vi "SquareFilter1.vi"(3 "error IN":errorcluster, 4 "Areas":dbl[][](array[numeric]), 5 "X,Y":dbl[][](array[numeric]), 6 "[IN] Chains (X,Y,dX,dY)":dbl[][](array[numeric])) -> (0 "error OUT":errorcluster, 2 "Filtered Chains (X,Y,dX,dY)":dbl[][](array[numeric]))   [LabVIEW 2013]
doc: "This simple filter cuts out displacement which connects particles with relative difference in areas more than 50%"
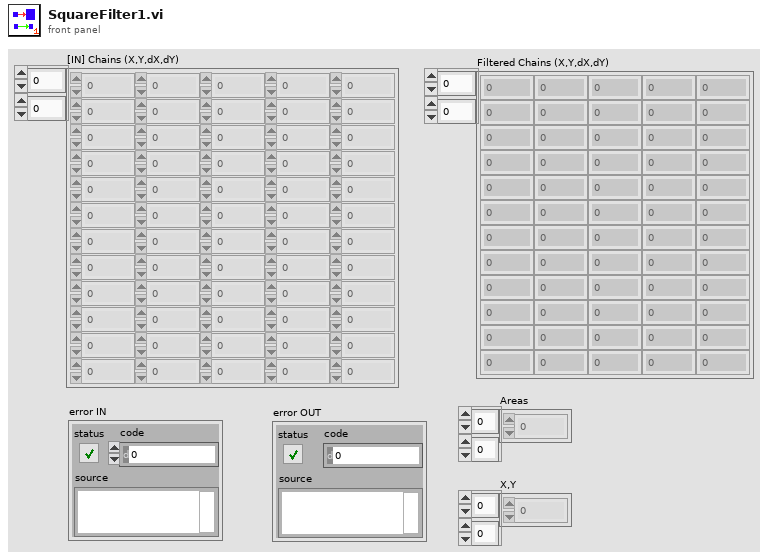
[diagram p1: front panel]
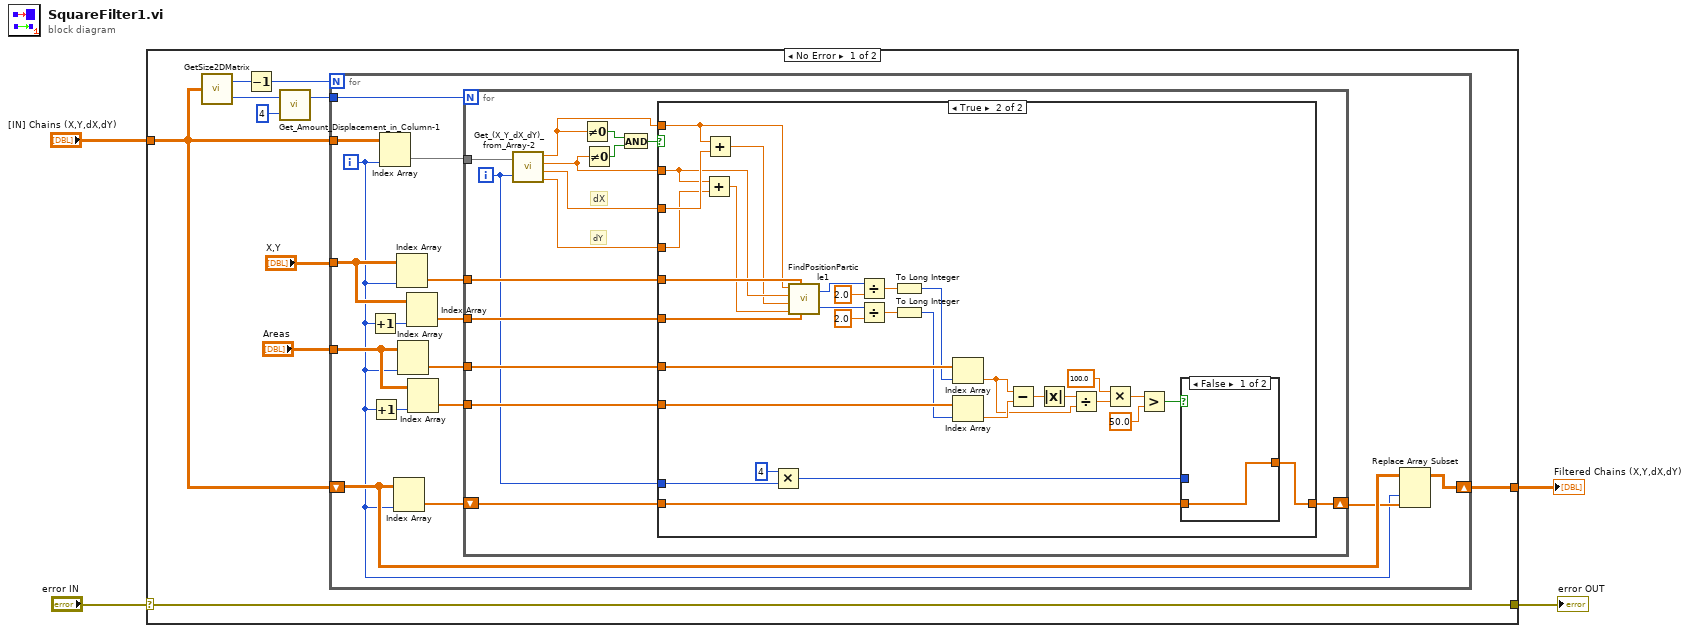
[diagram p0: block diagram]
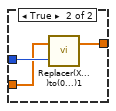
[diagram p3: hidden frame]
diagram:
  n1 = case shown="No Error" "error IN" {
    selector: "error IN" -> [w5 w83]
    tunnel: [w14 w84] -> w4
    tunnel: "[IN] Chains (X,Y,dX,dY)" -> [w10 w84]
    tunnel: [w5 w83] -> w1
    frame No Error {
      n2 = call "GetSize2DMatrix.vi"("Array IN (2D)"=w10) -> ("# Cols"=w9:i32, "# Rows"=w7:i32)
      n3 = Decrement(x=w9) -> (x-1=w13:i32)
      n4 = call "Get_Amount_Displacement_in_Column-1.vi"("multiplier"=4, "# Rows"=w7) -> ("Displ amount"=w6:i32)  [unwired: 1 out]
      n5 = for {
        N: w13 -> [_]
        tunnel: w10 -> [w29]
        shift-right: [w17] -> w14
        shift-left: w10 -> [w19]
        tunnel: "Areas" -> [w23]
        tunnel: "X,Y" -> [w28]
        tunnel: w6 -> [w15]
        i -> [w16]
        n6 = Increment(x=w16) -> (x+1=w27:i32)
        n7 = Increment(x=w16) -> (x+1=w24:i32)
        n8 = Index Array(array=w29, index (col)=w16) -> (element=w30:dbl[])  [unwired: 1 in]
        n9 = Index Array(array=w19, index (col)=w16) -> (element=w20:dbl[])  [unwired: 1 in]
        n10 = Index Array(array=w28, index (col)=w16) -> (element=w26:dbl[])  [unwired: 1 in]
        n11 = Index Array(array=w23, index (col)=w16) -> (element=w22:dbl[])  [unwired: 1 in]
        n12 = Index Array(array=w28, index (col)=w27) -> (element=w25:dbl[])  [unwired: 1 in]
        n13 = Index Array(array=w23, index (col)=w24) -> (element=w21:dbl[])  [unwired: 1 in]
        n14 = for {
          N: w15 -> [_]
          tunnel: w30 -> [w36]
          tunnel: w26 -> [w42]
          tunnel: w25 -> [w41]
          tunnel: w22 -> [w40]
          tunnel: w21 -> [w39]
          shift-right: [w37] -> w18
          shift-left: w20 -> [w38]
          i -> [w31]
          # "dY"
          # "dX"
          n15 = call "Get_(X_Y_dX_dY)_from_Array-2.vi"("(X,Y,dX,dY)"=w36, "Index of Displacement"=w31) -> ("X"=w35:dbl, "Y"=w34:dbl, "dX"=w33:dbl, "dY"=w32:dbl)
          n16 = Not Equal To 0?(x=w35) -> (x != 0?=w45:bool)
          n17 = Not Equal To 0?(x=w34) -> (x != 0?=w44:bool)
          n18 = And(x=w45, y=w44) -> (x .and. y?=w43:bool)
          n19 = case shown="True" w43 {
            tunnel: w34 -> [_ w73]
            tunnel: w35 -> [_ w74]
            tunnel: w33 -> [_ w78]
            tunnel: w32 -> [_ w77]
            tunnel: w42 -> [_ w76]
            tunnel: w41 -> [_ w75]
            tunnel: w40 -> [_ w66]
            tunnel: w39 -> [_ w62]
            tunnel: w38 -> [w46 w51]
            tunnel: [w46 w50] -> w37
            tunnel: w31 -> [_ w48]
            frame False {
            }
            frame True {
              n20 = Add(x=w73, y=w77) -> (x+y=w71:dbl)
              n21 = Add(x=w74, y=w78) -> (x+y=w72:dbl)
              n22 = Multiply(x=4, y=w48) -> (x*y=w47:i32)
              n23 = call "FindPositionParticle1.vi"("X,Y (2Frame)"=w75, "X,Y (1Frame)"=w76, "Y2"=w71, "X2"=w72, "Y1"=w73, "X1"=w74) -> ("Index X2"=w67:i32, "Index X1"=w69:i32)
              n24 = Divide(x=w69, y=2.0) -> (x/y=w65:dbl)
              n25 = Divide(x=w67, y=2.0) -> (x/y=w64:dbl)
              n26 = To Long Integer(number=w65) -> (32bit integer=w63:i32)
              n27 = To Long Integer(number=w64) -> (32bit integer=w61:i32)
              n28 = Index Array(array=w66, index=w63) -> (element=w57:dbl)
              n29 = Index Array(array=w62, index=w61) -> (element=w60:dbl)
              n30 = Subtract(x=w57, y=w60) -> (x-y=w59:dbl)
              n31 = Absolute Value(x=w59) -> (abs(x)=w58:dbl)
              n32 = Divide(x=w58, y=w57) -> (x/y=w56:dbl)
              n33 = Multiply(x=100.0, y=w56) -> (x*y=w54:dbl)
              n34 = Greater?(x=w54, y=50.0) -> (0:w52:bool)
              n35 = case shown="False" w52 {
                tunnel: w51 -> [w79 w81]
                tunnel: w47 -> [_ w82]
                tunnel: [w79 w80] -> w50
                frame False {
                }
                frame True {
                  n36 = call "Replacer(X...)to(0...)1.vi"("[IN] Starting index"=w82, "[IN] Array"=w81) -> ("Replaced array"=w80:dbl[])  [unwired: 1 out]
                }
              }
            }
          }
        }
        n37 = Replace Array Subset(array=w19, new element=w18, index (col)=w16) -> (w17:dbl[][])  [unwired: 1 in]
      }
    }
    frame Error {
    }
  }
  "error OUT" <- w1
  "Filtered Chains (X,Y,dX,dY)" <- w4
